vi "MQTT_ConnAck_Read.vi"(8 "error in (no error)":errorcluster, 11 "SSL_Connection":T1) -> (0 "error out":errorcluster, 1 "QoS Level":T3, 2 "Connection Status":T2=enum."Connection refused: not authorized", 3 "SSL_Connection 2":T1, 5 "MessageType":T4)   [LabVIEW 2015, in "MQTT_Functions.lvlib"]
doc: "This VI processes the connection acknowledge message from the server.\n\n© 2015 - daq.io, LLC - Peter Adelhardt"
uses:
  MQTT_Functions.lvlib
  Controls/MessageType.ctl
  Controls/QoS.ctl
  Controls/Connection_Return_Codes.ctl
  AWS-IoT-RESTful/Controls/SSL_Connection.ctl
  AWS-IoT-RESTful/AWS_IoT.lvlib
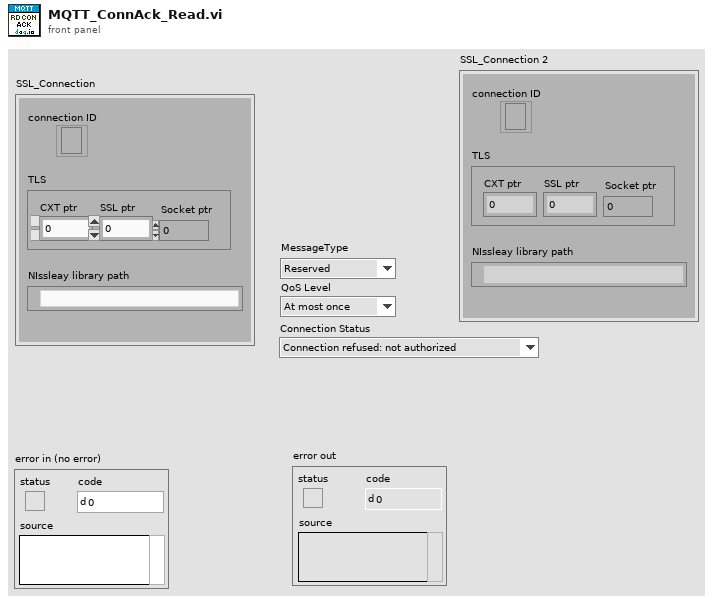
[diagram p1: front panel]
types:
  T1 = typedef "AWS_IoT.lvlib/SSL_Connection.ctl" = cluster{"connection ID":refnum<k5>, "TLS":cluster{"CXT ptr":i32, "SSL ptr":i32, "Socket ptr":u64}, "NIssleay library path":path}
  T2 = typedef "MQTT_Functions.lvlib/Connection_Return_Codes.ctl" = enum16{"Connection accepted", "Connection refused: unacceptable protocol version", "Connection refused: identifier rejected", "Connection refused: Server unavailable", "Connection refused: bad user name or password", "Connection refused: not authorized"}
  T3 = typedef "MQTT_Functions.lvlib/QoS.ctl" = enum8{"At most once", "At least once", "Exactly once", "Reserved"}
  T4 = typedef "MQTT_Functions.lvlib/MessageType.ctl" = enum32{"Reserved", "CONNECT", "CONNACK", "PUBLISH", "PUBACK", "PUBREC", "PUBREL", "PUBCOMP", "SUBSCRIBE", "SUBACK", "UNSUBSCRIBE", "UNSUBACK", "PINGREQ", "PINGRESP", "DISCONNECT", "Reserved2"}
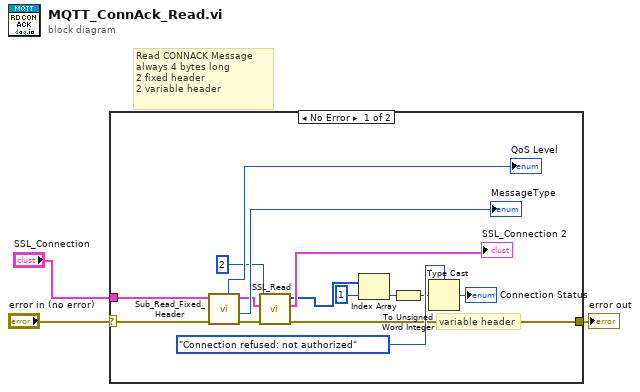
[diagram p0: block diagram]
diagram:
  # "Read CONNACK Message\nalways 4 bytes long\n2 fixed header\n2 variable header"
  n1 = case shown="No Error" "error in (no error)" {
    selector: "error in (no error)" -> [w16 w19]
    tunnel: [w9 w19] -> w2
    tunnel: "SSL_Connection" -> [w7 _]
    frame No Error {
      # "variable header"
      n2 = call "Sub_Read_Fixed_Header.vi"("error in (no error)"=w16, "SSL_Connection"=w7) -> ("error out"=w10:errorcluster, "MessageType"=→"MessageType":T4, "SSL_Connection 2"=w5:T1, "QoS Level"=→"QoS Level":T3)  [unwired: 3 in, 3 out]
      n3 = call "SSL_Read.vi"("error in (no error)"=w10, "SSL_Connection"=w5, "bytes to read"=2) -> ("error out"=w9:errorcluster, "SSL_Connection 2"=→"SSL_Connection 2":T1, "data out"=w4:u8[])  [unwired: 6 in]
      n4 = Index Array(array=w4, index=1) -> (element=w18:u8)
      n5 = To Unsigned Word Integer(number=w18) -> (unsigned 16bit integer=w8:u16)
      n6 = Type Cast(type=Connection_Return_Codes."Connection refused: not authorized" ("Conn Return Code"), x=w8) -> (*(type *) &x=→"Connection Status":T2)
    }
    frame Error {
    }
  }
  "error out" <- w2
